vi "Get SystemLink Server Configured for Local System.vi"(8 "error in (no error)":errorcluster) -> (0 "error out":errorcluster, 3 "SystemLink Server Configured for Local System":string)   [LabVIEW 2017]
uses:
  <vilib>/Utility/sysdir.llb/System Directory Type.ctl
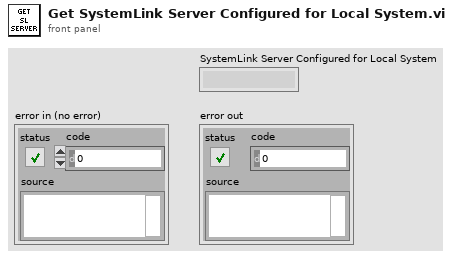
[diagram p1: front panel]
types:
  T1 = typedef "System Directory Type.ctl" = i32
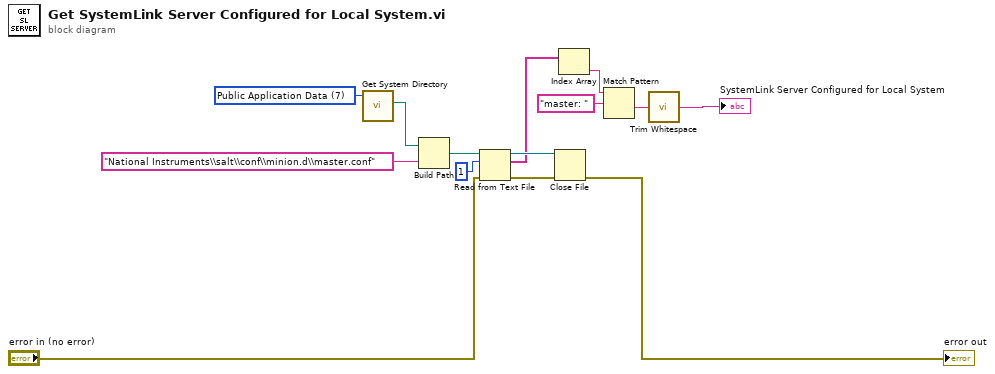
[diagram p0: block diagram]
diagram:
  w4 = T1 7 items=["User Home"=0, "User Desktop"=1, "User Documents"=2, "User Application Data"=3, "User Preferences"=4, "User Temporary"=5, "Public Documents"=6, "Public Application Data"=7, "Public Preferences"=8, "Public Cache"=13, "System Core Libraries"=9, "System Installed Libraries"=10, "Application Files"=11, "Boot Volume Root"=12] ("system directory type")
  n1 = call <vilib>:"Get System Directory.vi"("system directory type"=w4) -> ("system directory"=w12:path)  [unwired: 10 in]
  n2 = Build Path(base path=w12, name or relative path="National Instruments\\salt\\conf\\minion.d\\master.conf") -> (appended path=w6:path)
  n3 = Read from Text File(file (use dialog)=w6, count=1, error in="error in (no error)") -> (refnum out=w13:refnum<file>, text=w8:string[], error out=w14:errorcluster)  [unwired: 1 in, 1 out]
  n4 = Close File(refnum=w13, error in=w14) -> (error out=→"error out":errorcluster)  [unwired: 1 out]
  n5 = Index Array(array=w8) -> (element=w9:string)  [unwired: 1 in]
  n6 = Match Pattern(string=w9, regular expression="master: ") -> (after substring=w11:string)  [unwired: 1 in, 3 out]
  n7 = call <vilib>:"Trim Whitespace.vi"("string"=w11) -> ("trimmed string"=→"SystemLink Server Configured for Local System":string)  [unwired: 1 in]
